vi "sec_AlarmLogic_main.vi"(7 "Command":T3=enum."Set Alarm Switches", 8 "error in (no error)":errorcluster, 9 "Tamper Switches":bool[](array[boolean]), 10 "Bypass Switches":bool[](array[boolean]), 11 "Alarm Switches":bool[](array[boolean])) -> (0 "error out":errorcluster, 3 "Alarm States":T1[](array[typedef]))   [LabVIEW 2009]
doc: "This module is responsible for determining the Alarm State.\nSee block diagram for Alarm Logic details."
uses:
  sec_AlarmLogic_Command_enum.ctl
  sec_AlarmLogic_State_cluster.ctl
  controls/sec_AlarmStates_enum.ctl
panel:
  in  "State (type)":T2
  # "Inputs"
  # "Outputs"
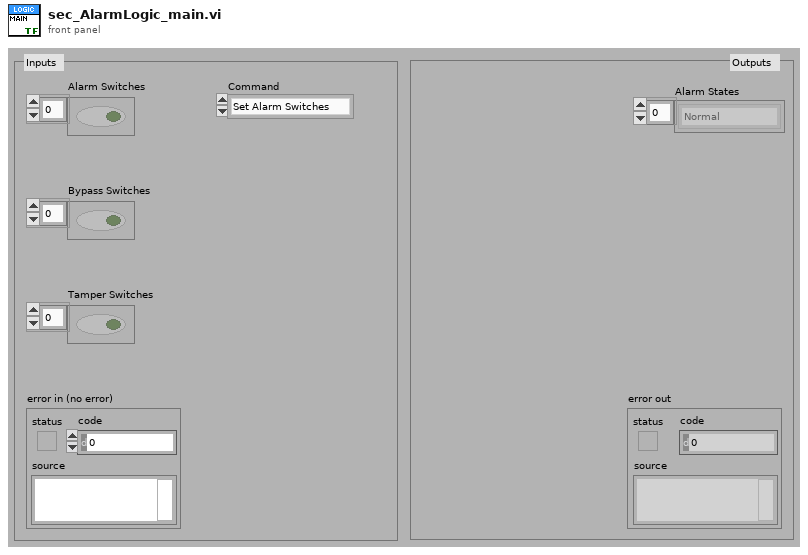
[diagram p1: front panel]
types:
  T1 = typedef "sec_AlarmStates_enum.ctl" = enum16{"Normal", "Alarm", "Bypass", "Tamper"}
  T2 = typedef "sec_AlarmLogic_State_cluster.ctl" = cluster{"Alarm Switches":bool[], "Bypass Switches":bool[], "Tamper Switches":bool[], "Alarm Status":bool[], "Alarm States":T1[]}
  T3 = typedef "sec_AlarmLogic_Command_enum.ctl" = enum16{"Initialise", "Set Alarm Switches", "Check Alarm States", "Get Alarm States"}
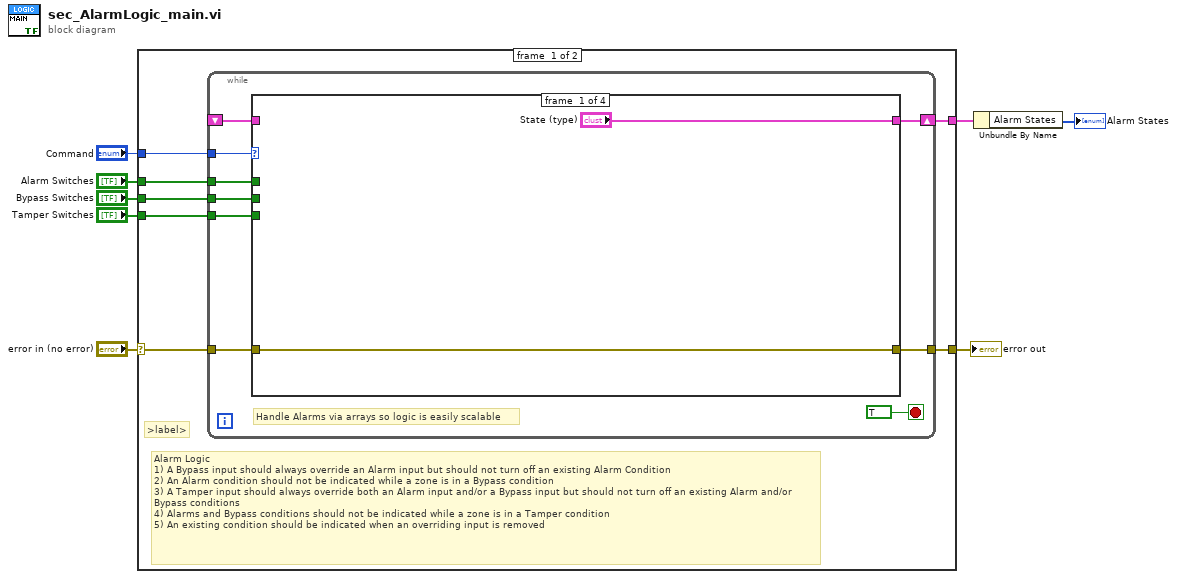
[diagram p0: block diagram]
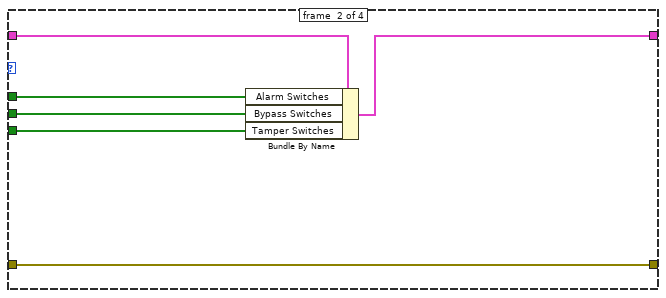
[diagram p2: hidden frame]
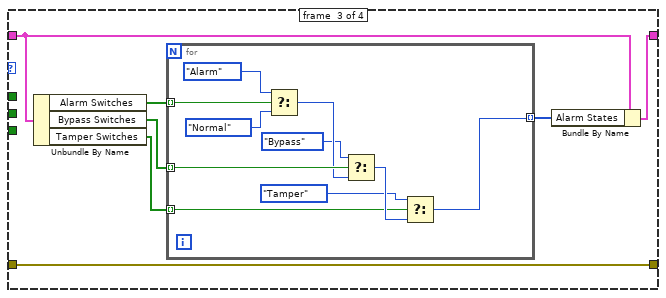
[diagram p3: hidden frame]
diagram:
  n1 = case shown="No Error" "error in (no error)" {
    selector: "error in (no error)" -> [w10 w52]
    tunnel: [w9 w52] -> w7
    tunnel: "Command" -> [w11 _]
    tunnel: "Alarm Switches" -> [w15 _]
    tunnel: "Bypass Switches" -> [w14 _]
    tunnel: "Tamper Switches" -> [w13 _]
    tunnel: [w12 _] -> w2
    frame #0 {
      # "Alarm Logic\n1) A Bypass input should always override an Alarm input but should not turn off an existing Alarm Condition\n2) An Alarm condition should not be indicated while a zone is in a Bypass condition\n3) A Tamper input should always override both an Alarm input and/or a Bypass input but should not turn off an existing Alarm and/or Bypass conditions\n4) Alarms and Bypass conditions should not be indicated while a zone is in a Tamper condition\n5) An existing condition should be indicated when an overriding input is removed"
      # ">label>"
      n2 = while {
        tunnel: w15 -> [w24]
        tunnel: w14 -> [w23]
        tunnel: w13 -> [w22]
        shift-right: [w21] -> w12
        shift-left: _ -> [w20]
        tunnel: w11 -> [w18]
        tunnel: w10 -> [w17]
        tunnel: [w16] -> w9
        stop <- TRUE stop-if-true
        # "Handle Alarms via arrays so logic is easily scalable"
        n3 = case shown="\"Get Alarm States\"" w18 {
          tunnel: w24 -> [_ w30 _ _]
          tunnel: w23 -> [_ w29 _ _]
          tunnel: w22 -> [_ w28 _ _]
          tunnel: ["State (type)" w31 w37 w51] -> w21
          tunnel: w20 -> [_ w32 w39 w51]
          tunnel: w17 -> [w25 w27 w38 w50]
          tunnel: [w25 w27 w38 w50] -> w16
          frame #0 {
          }
          frame #1 {
            n4 = Bundle By Name(cluster=w32, "Alarm Switches"=w30, "Bypass Switches"=w29, "Tamper Switches"=w28) -> (w31:T2)
          }
          frame #2 {
            n5 = Unbundle By Name(w39) -> ("Alarm Switches"=w36:bool[], "Bypass Switches"=w35:bool[], "Tamper Switches"=w34:bool[])
            n6 = for {
              tunnel: w36 -> [w48] mode=indexing
              tunnel: w35 -> [w49] mode=indexing
              tunnel: w34 -> [w41] mode=indexing
              tunnel: [w40] -> w33 mode=indexing
              n7 = Select(t=sec_AlarmStates_enum."Alarm" ("Alarm State"), s=w48, f=sec_AlarmStates_enum."Normal" ("Alarm State")) -> (s? t:f=w45:T1)
              n8 = Select(t=sec_AlarmStates_enum."Bypass", s=w49, f=w45) -> (s? t:f=w43:T1)
              n9 = Select(t=sec_AlarmStates_enum."Tamper", s=w41, f=w43) -> (s? t:f=w40:T1)
            }
            n10 = Bundle By Name(cluster=w39, "Alarm States"=w33) -> (w37:T2)
          }
          frame #3 {
          }
        }
      }
    }
    frame #1 {
    }
  }
  "error out" <- w7
  n11 = Unbundle By Name(w2) -> ("Alarm States"=→"Alarm States":T1[])
